vi "Robocopy Current Backup.vi"(6 "Dest. drive root":path=path "S:/Research/EnFlo_Data", 7 "Source drive root":path=path "S:/Research/EnFlo_Data_Current") -> (0 "Errors out":errorcluster[](array[cluster]), 1 "Commands":string[](array[string]), 3 "End summary":string[](array[string]))   [LabVIEW 2020]
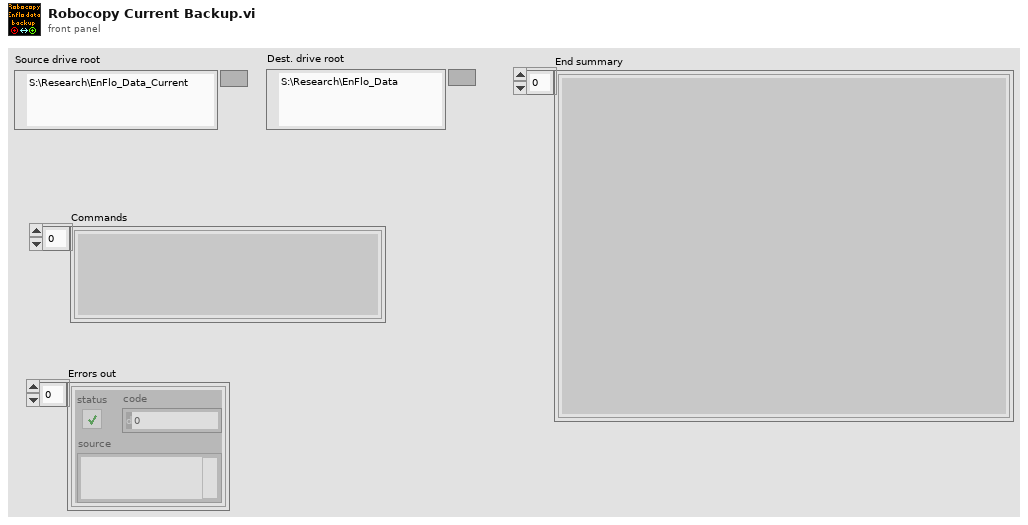
[diagram p1: front panel]
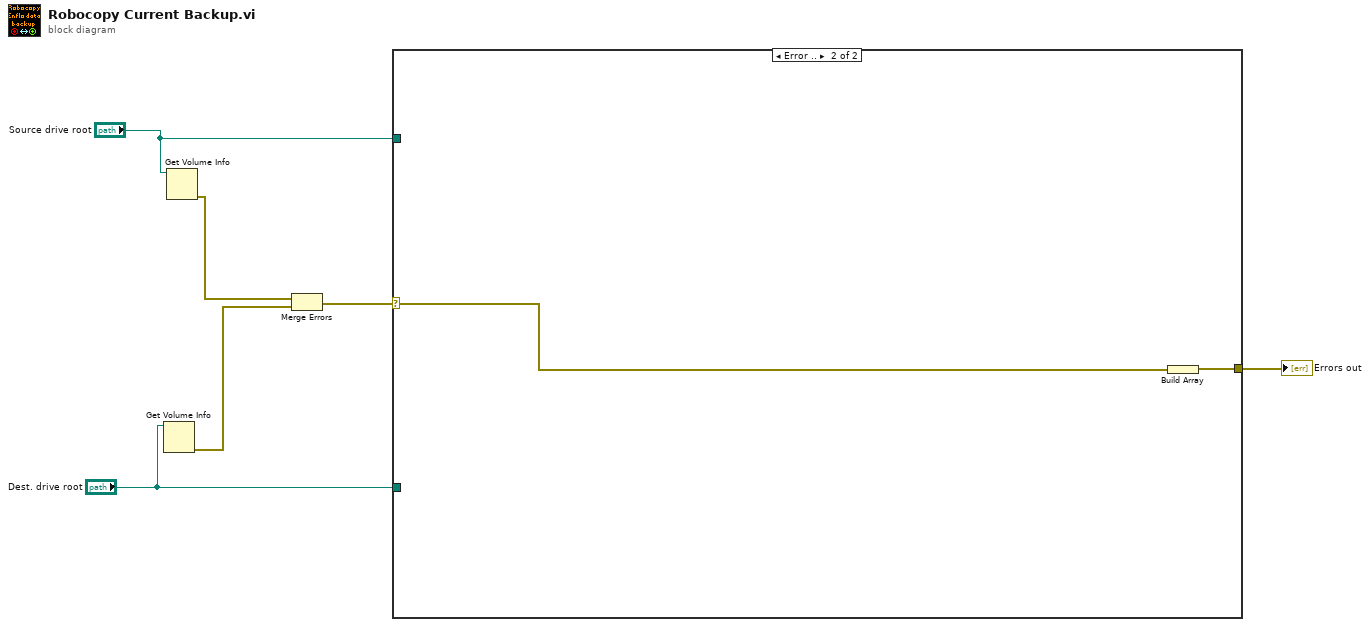
[diagram p0: block diagram]
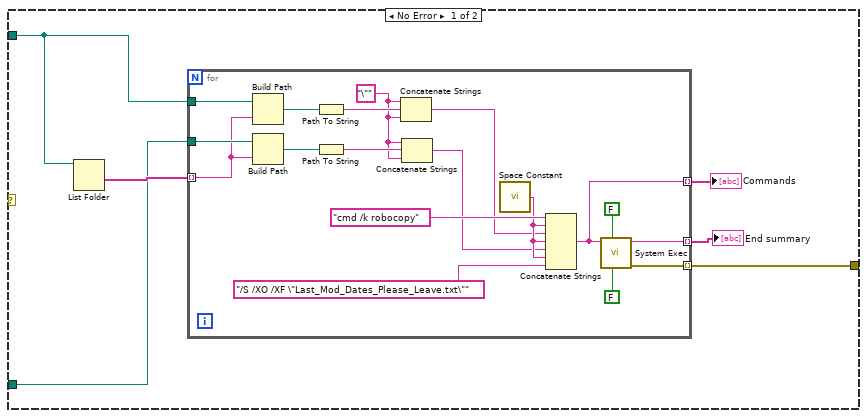
[diagram p2: hidden frame]
diagram:
  n1 = Get Volume Info(11:"Dest. drive root") -> (0:w2:errorcluster)  [unwired: 1 in, 5 out]
  n2 = Get Volume Info(11:"Source drive root") -> (0:w3:errorcluster)  [unwired: 1 in, 5 out]
  n3 = Merge Errors(w3, w2) -> (w1:errorcluster)
  n4 = case shown="Error .." w1 {
    selector: w1 -> [_ w32]
    tunnel: [w12 w31] -> w6
    tunnel: "Source drive root" -> [w8 _]
    tunnel: "Dest. drive root" -> [w7 _]
    frame No Error {
      n5 = List Folder(path=w8) -> (folder names=w9:string[])  [unwired: 3 in, 3 out]
      n6 = for {
        tunnel: w8 -> [w28]
        tunnel: w7 -> [w27]
        tunnel: w9 -> [w26] mode=indexing
        tunnel: [w21] -> w12 mode=indexing
        tunnel: [w14] -> w11 mode=indexing
        tunnel: [w13] -> w10 mode=indexing
        w15 = "\"" ("string")
        n7 = Build Path(base path=w28, name or relative path=w26) -> (appended path=w24:path)
        n8 = Build Path(base path=w27, name or relative path=w26) -> (appended path=w23:path)
        n9 = Path To String(path=w24) -> (string=w19:string)
        n10 = Path To String(path=w23) -> (string=w17:string)
        n11 = Concatenate Strings(w15, w19, w15) -> (w18:string)
        n12 = Concatenate Strings(w15, w17, w15) -> (w16:string)
        n13 = call <vilib>:"Space Constant.vi"() -> ("String"=w20:string)
        n14 = Concatenate Strings("cmd /k robocopy", w20, w18, w20, w16, w20, "/S /XO /XF \"Last_Mod_Dates_Please_Leave.txt\"" ("string")) -> (w14:string)
        n15 = call <vilib>:"System Exec.vi"("run minimized? (F)"=FALSE, "wait until completion? (T)"=FALSE, "command line"=w14) -> ("error out"=w21:errorcluster, "standard output"=w13:string)  [unwired: 5 in, 2 out]
      }
      "Commands" <- w11
      "End summary" <- w10
    }
    frame Error {
      n16 = Build Array(w32) -> (w31:errorcluster[])
    }
  }
  "Errors out" <- w6
